vi "Arm Controller.vi"(8 "error in":errorcluster) -> ()   [LabVIEW 2018]
doc: "This VI executes continuously carrying out the current operation and responding to updates or new operations. It will often contain the timing or control code that is difficult to place directly in TeleOp. This VI generally opens all sensors and motors and isolates the rest of the robot code from knowing how the operations are carried out."
uses:
  <vilib>/Rock Robotics/WPI/Framework/Completion Status.ctl
  Arm Setpoints.ctl
  Arm Operations.ctl
  <vilib>/Rock Robotics/WPI/ThirdParty/Phoenix-LabVIEW/Motor Controller/Controls/CTRE_Phoenix_MotorControl_FeedbackDevice.ctl
  <vilib>/Rock Robotics/WPI/ThirdParty/Phoenix-LabVIEW/Motor Controller/Controls/CTRE_Phoenix_MotorControl_LimitSwitchSource_Local.ctl
  <vilib>/Rock Robotics/WPI/ThirdParty/Phoenix-LabVIEW/Motor Controller/Controls/CTRE_Phoenix_MotorControl_LimitSwitchNormal.ctl
  <vilib>/Rock Robotics/WPI/ThirdParty/Phoenix-LabVIEW/Motor Controller/Controls/CTRE_Phoenix_MotorControl_StatusFrameEnhanced.ctl
  <vilib>/Rock Robotics/WPI/ThirdParty/Phoenix-LabVIEW/Motor Controller/Controls/CTRE_Phoenix_MotorControl_VelocityMeasurementPeriod.ctl
  <vilib>/Rock Robotics/WPI/ThirdParty/Phoenix-LabVIEW/Motor Controller/Controls/CTRE_Phoenix_MotorControl_ControlMode.ctl
  <extravilib>/ChannelInstances/Lossy Stream-c(i32,i32,i32,i32)/Write With Abort.vi
  <extravilib>/ChannelInstances/Lossy Stream-c(i32,i32,i32,i32)/Read With Abort.vi
  <extravilib>/ChannelInstances/Lossy Stream-c(i32,i32,i32,i32)/Endpoint.vi
  <extravilib>/ChannelInstances/Lossy Stream-c(i32,i32,i32,i32)/EndpointRead.vi
  <extravilib>/ChannelInstances/Lossy Stream-c(i32,i32,i32,i32)/Instantiate.vi
  <extravilib>/ChannelInstances/Lossy Stream-c(i32,i32,i32,i32)/)Channel.vi
  <resource>/ChannelSupport/_ChannelSupport/WaitIfNeeded.vi
  <vilib>/Rock Robotics/WPI/ThirdParty/Phoenix-LabVIEW/Motor Controller/Get/CTRE_Phoenix_MotorController_GetSelectedSensorData.vi
  <extravilib>/ChannelInstances/Lossy Stream-c(i32,i32,i32,i32).lvlib
  <vilib>/Rock Robotics/Network Tables/NT Write Boolean.vi
panel:
  in  "F":dbl=11.9
  in  "D":dbl
  in  "I":dbl
  in  "P":dbl=8.0
  in  "Acceleration":i32=120
  in  "Cruise Velocity":i32=40
  in  "Gravity Compensator":dbl=0.038 format="%#_13g"
  in  "Interactive Values":T1
  out "Current\nCmd":string
  in  "Buttons":cluster{"Execute Cmd":bool, "Abort Cmd":bool}
  out "Command Timing":cluster{"Start Time (ms)":u32, "Iterations":i32}
  out "Status":T3
  # "Tip: It may be helpful to observe inputs and sensor values.\nYou may also want to display tuning or debugging controls."
  # "Interactive Command: You may fill in the settings for a command\nand schedule it with the Execute button. You can observe and abort\nany command while fine tuning the code for the controller."
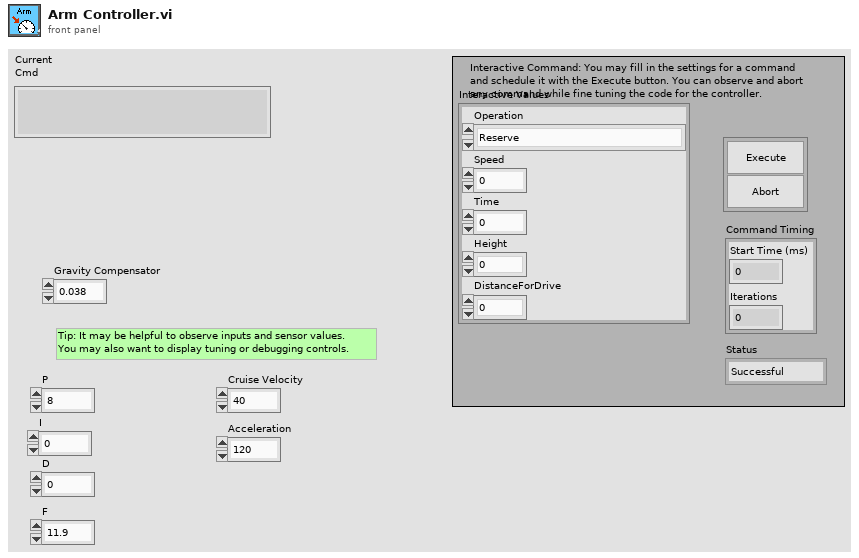
[diagram p1: front panel]
types:
  T1 = typedef "Arm Setpoints.ctl" = cluster{"Operation":T2, "Speed":dbl, "Time":dbl, "Height":dbl, "DistanceForDrive":dbl}
  T2 = typedef "Arm Operations.ctl" = enum16{"Reserve", "Read Current", "Immediate", "RaiseForTime", "GoToHeight", "StayAtHeight", "RaiseAfterTime", "RaiseAfterDriveAtDistance"}
  T3 = typedef "Completion Status.ctl" = enum16{"Successful", "Aborted", "Incomplete"}
  T4 = typedef "CTRE_Phoenix_MotorControl_VelocityMeasurementPeriod.ctl" = u16
  T5 = typedef "CTRE_Phoenix_MotorControl_StatusFrameEnhanced.ctl" = u16
  T6 = typedef "CTRE_Phoenix_MotorControl_LimitSwitchNormal.ctl" = enum16{"Normally Open", "Normally Closed", "Disabled"}
  T7 = typedef "CTRE_Phoenix_MotorControl_LimitSwitchSource_Local.ctl" = enum16{"Feedback Connector", "Remote Talon SRX", "Remote CANifier", "Deactivated"}
  T8 = typedef "CTRE_Phoenix_MotorControl_FeedbackDevice.ctl" = i8
  T9 = typedef "WPI_MotorControlDeviceRef.ctl" = cluster{"DeviceStatus":errorcluster, "Type":T10, "PWM":cluster{"PWM Channel":T11, "DeadBand":T12}, "CAN":cluster{"Device Number":u8, "SetOutput VI Ref":variant, "GetOutput VI Ref":variant, "Enable VI Ref":variant, "Disable VI Ref":variant, "Data":variant}, "Invert":bool, "DIO PWM":cluster{"PWM \"Enable\" Channel":T11, "DIOChannel":T13, "PWM Rate":dbl}}
  T10 = typedef "WPI_MotorControlType.ctl" = enum16{"PWM", "CAN", "DIO PWM"}
  T11 = typedef "FPGA_DIOPWMChannel.ctl" = enum8{"PWM 0", "PWM 1", "PWM 2", "PWM 3", "PWM 4", "PWM 5", "PWM 6", "PWM 7", "PWM 8", "PWM 9", "PWM MXP 0", "PWM MXP 1", "PWM MXP 2", "PWM MXP 3", "PWM MXP 4", "PWM MXP 5", "PWM MXP 6", "PWM MXP 7", "PWM MXP 8", "PWM MXP 9", "Invalid"}
  T12 = typedef "WPI_PWMDeadband.ctl" = cluster{"Name":string, "maxPositivePwm":i32, "minPositivePwm":i32, "centerPwm":i32, "maxNegativePwm":i32, "minNegativePwm":i32, "angularRange":u16}
  T13 = typedef "FPGA_DIOChannel.ctl" = enum8{"DIO 0", "DIO 1", "DIO 2", "DIO 3", "DIO 4", "DIO 5", "DIO 6", "DIO 7", "DIO 8", "DIO 9", "DIO MXP 0", "DIO MXP 1", "DIO MXP 2", "DIO MXP 3", "DIO MXP 4", "DIO MXP 5", "DIO MXP 6", "DIO MXP 7", "DIO MXP 8", "DIO MXP 9", "DIO MXP 10", "DIO MXP 11", "DIO MXP 12", "DIO MXP 13", "DIO MXP 14", "DIO MXP 15", "SPI Port CS1", "SPI Port CS2", "SPI Port CS3", "SPI Port MISO", "SPI Port MOSI", "Invalid"}
  T14 = typedef "Command Status Info.ctl" = cluster{"Name":string, "Status":T3, "notifier out":T15}
  T15 = typedef "Completion Notifier.ctl" = refnum<notifier>
  T16 = cluster{"Current Command":T1, "Command Timing":cluster{"Start Time (ms)":u32, "Iterations":i32}, "Command Arguments":cluster{"Command Info":T14, "Description":string, "Default Command":T1, "queue out":refnum<queue>, "Subsystem Name":string}}
  T17 = cluster{"Position":i32, "Velocity":i32, "Target Position":i32, "Target Velocity":i32}
  T18 = typedef "Lossy Stream-c(i32,i32,i32,i32).lvlib/)Channel.ctl" = refnum<queue>
  T19 = enum16{"DemandType_Neutral", "DemandType_AuxPID", "DemandType_ArbitraryFeedForward"}
  T20 = cluster{"Operation":T2, "Height":dbl, "DistanceForDrive":dbl, "Time":dbl}
  T21 = typedef "CTRE_Phoenix_MotorControl_ControlMode.ctl" = u16
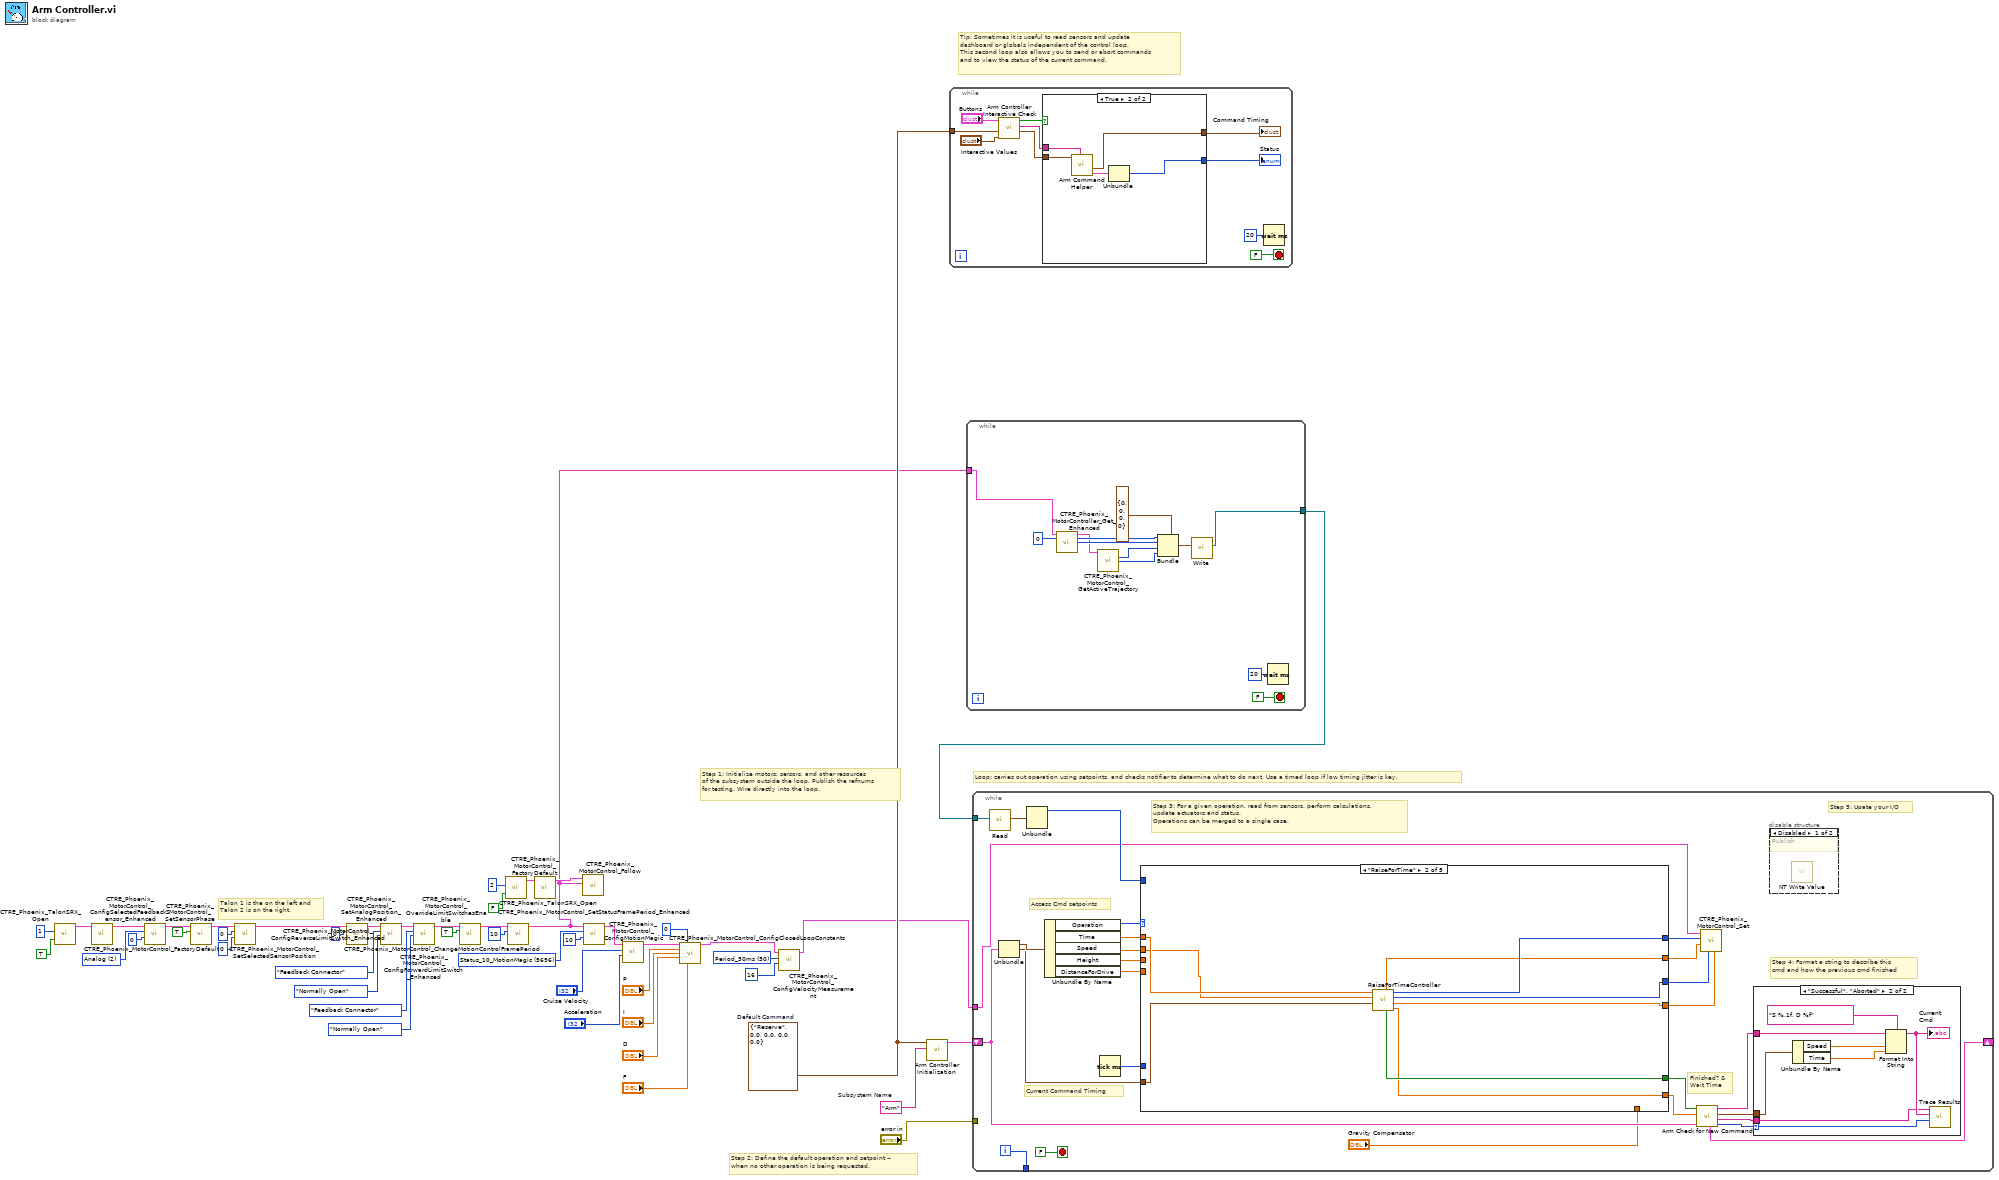
[diagram p0: block diagram]
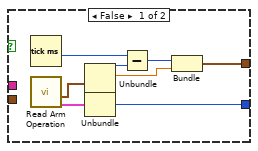
[diagram p2: hidden frame]
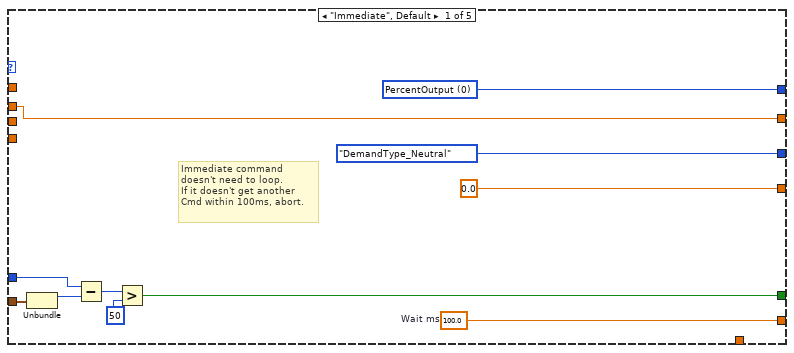
[diagram p5: hidden frame]
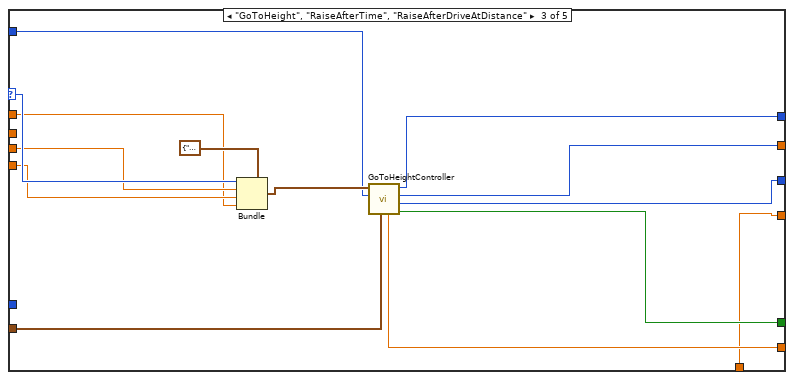
[diagram p6: hidden frame]
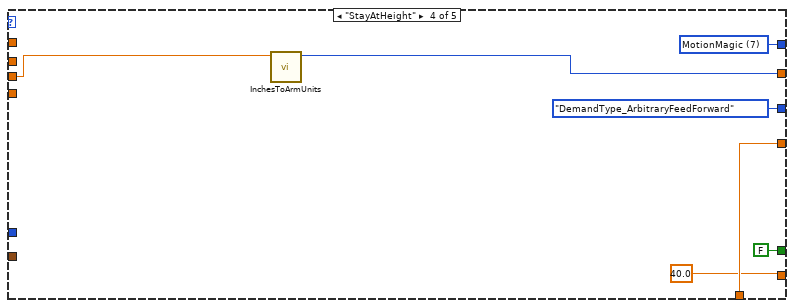
[diagram p7: hidden frame]
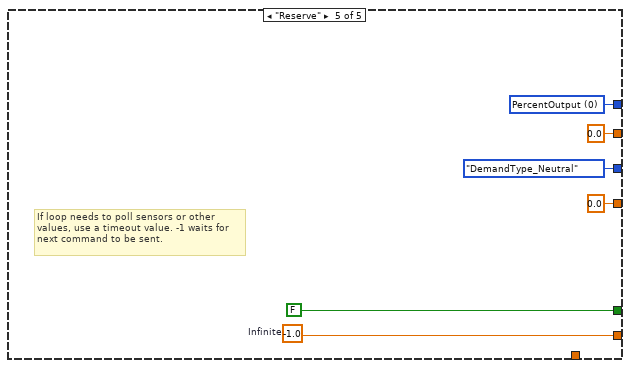
[diagram p8: hidden frame]
diagram:
  w13 = T4 50 items=["Period_1ms"=1, "Period_2ms"=2, "Period_5ms"=5, "Period_10ms"=10, "Period_20ms"=20, "Period_25ms"=25, "Period_50ms"=50, "Period_100ms"=100] ("Velocity Measurement Period")
  w21 = T5 5696 items=["Status_1_General"=5120, "Status_2_Feedback0"=5184, "Status_3_Quadrature"=5248, "Status_4_AinTempVbat"=5312, "Status_6_Misc"=5440, "Status_7_CommStatus"=5504, "Status_8_PulseWidth"=5568, "Status_9_MotProfBuffer"=5632, "Status_10_MotionMagic"=5696, "Status_11_UartGadgeteer"=5760, "Status_12_Feedback1"=5824, "Status_13_Base_PIDF0"=5888, "Status_14_Turn_PIDF1"=5952, "Status_15_FirmwareApiStatus"=6016] ("Status Frame")
  w38 = T8 2 items=["QuadEncoder"=0, "Analog"=2, "Tachometer"=4, "Pulse Width Encoded Position"=8, "Sensor Sum (S0 + S1)"=9, "Sensor Difference (D0 - D1)"=10, "Remote Source 0"=11, "Remote Source 1"=12, "Software Emulated"=15] ("Feedback Device")
  w45 = T1 {"Operation"=enum."Reserve", "Speed"=0.0, "Time"=0.0, "Height"=0.0, "DistanceForDrive"=0.0}  # Default Command
  w46 = "Arm"  # Subsystem Name
  # "Talon 1 is the on the left and\nTalon 2 is on the right."
  # "Tip: Sometimes it is useful to read sensors and update\ndashboard or globals independent of the control loop.\nThis second loop also allows you to send or abort commands\nand to view the status of the current command."
  # "Step 2: Define the default operation and setpoint --\nwhen no other operation is being requested."
  # "Step 1: Initialize motors, sersors, and other resources\nof the subsystem outside the loop. Publish the refnums\nfor testing. Wire directly into the loop."
  # "Loop: carries out operation using setpoints, and checks notifier to determine what to do next. Use a timed loop if low timing jitter is key."
  n1 = call <vilib>:"CTRE_Phoenix_TalonSRX_Open.vi"("Invert"=TRUE, "Device Number"=u8 1) -> ("CAN Talon SRX Ref"=w42:T9)  [unwired: 8 in, 1 out]
  n2 = call <vilib>:"CTRE_Phoenix_MotorControl_FactoryDefault.vi"("PhoenixMotorControlDevRef"=w42) -> ("PhoenixMotorControlDevRef"=w39:T9)  [unwired: 9 in, 1 out]
  n3 = call <vilib>:"CTRE_Phoenix_MotorControl_ConfigSelectedFeedbackSensor_Enhanced.vi"("pidLoopIdx"=0, "Feedback Device"=w38, "PhoenixMotorControlDevRef"=w39) -> ("PhoenixMotorControlDevRef"=w26:T9)  [unwired: 7 in, 1 out]
  n4 = call <vilib>:"CTRE_Phoenix_MotorControl_SetSensorPhase.vi"("PhaseSensor"=TRUE, "PhoenixMotorControlDevRef"=w26) -> ("PhoenixMotorControlDevRef"=w24:T9)  [unwired: 8 in, 1 out]
  n5 = call <vilib>:"CTRE_Phoenix_MotorControl_SetSelectedSensorPosition.vi"("pidLoopIdx"=u32 0, "New Sensor Position"=0, "PhoenixMotorControlDevRef"=w24) -> ("PhoenixMotorControlDevRef"=w17:T9)  [unwired: 7 in, 1 out]
  n6 = call <vilib>:"CTRE_Phoenix_MotorControl_SetAnalogPosition_Enhanced.vi"("New Position"=0, "PhoenixMotorControlDevRef"=w17) -> ("PhoenixMotorControlDevRef"=w16:T9)  [unwired: 8 in, 1 out]
  n7 = call <vilib>:"CTRE_Phoenix_MotorControl_ConfigReverseLimitSwitch_Enhanced.vi"("PhoenixMotorControlDevRef"=w16, "Limit Switch Source"=CTRE_Phoenix_MotorControl_LimitSwitchSource_Local."Feedback Connector", "NormallyOpenOrClosed"=CTRE_Phoenix_MotorControl_LimitSwitchNormal."Normally Open") -> ("PhoenixMotorControlDevRef"=w34:T9)  [unwired: 11 in, 1 out]
  n8 = call <vilib>:"CTRE_Phoenix_MotorControl_ConfigForwardLimitSwitch_Enhanced.vi"("PhoenixMotorControlDevRef"=w34, "Limit Switch Source"=CTRE_Phoenix_MotorControl_LimitSwitchSource_Local."Feedback Connector", "NormallyOpenOrClosed"=CTRE_Phoenix_MotorControl_LimitSwitchNormal."Normally Open") -> ("PhoenixMotorControlDevRef"=w29:T9)  [unwired: 11 in, 1 out]
  n9 = call <vilib>:"CTRE_Phoenix_MotorControl_OverrideLimitSwitchesEnable.vi"("PhoenixMotorControlDevRef"=w29, "Override Limit Switch Enable?"=TRUE) -> ("PhoenixMotorControlDevRef"=w19:T9)  [unwired: 12 in, 1 out]
  n10 = call <vilib>:"CTRE_Phoenix_TalonSRX_Open.vi"("Invert"=FALSE, "Device Number"=u8 2) -> ("CAN Talon SRX Ref"=w40:T9)  [unwired: 8 in, 1 out]
  n11 = call <vilib>:"CTRE_Phoenix_MotorControl_ChangeMotionControlFramePeriod.vi"("periodMs"=10, "PhoenixMotorControlDevRef"=w19) -> ("PhoenixMotorControlDevRef"=w2:T9)  [unwired: 8 in, 1 out]
  n12 = call <vilib>:"CTRE_Phoenix_MotorControl_FactoryDefault.vi"("PhoenixMotorControlDevRef"=w40) -> ("PhoenixMotorControlDevRef"=w27:T9)  [unwired: 9 in, 1 out]
  n13 = call <vilib>:"CTRE_Phoenix_MotorControl_Follow.vi"("Master Controller to Follow"=w2, "PhoenixMotorControlDevRef"=w27) -> ()  [unwired: 8 in, 2 out]
  n14 = call <vilib>:"CTRE_Phoenix_MotorControl_SetStatusFramePeriod_Enhanced.vi"("periodMs"=10, "Status Frame"=w21, "PhoenixMotorControlDevRef"=w2) -> ("PhoenixMotorControlDevRef"=w4:T9)  [unwired: 7 in, 1 out]
  n15 = call <vilib>:"CTRE_Phoenix_MotorControl_ConfigMotionMagic.vi"("Acceleration"="Acceleration", "Cruise Velocity"="Cruise Velocity", "PhoenixMotorControlDevRef"=w4) -> ("PhoenixMotorControlDevRef"=w7:T9)  [unwired: 7 in, 1 out]
  n16 = call <vilib>:"CTRE_Phoenix_MotorControl_ConfigClosedLoopConstants.vi"("PhoenixMotorControlDevRef"=w7, "slotIdx"=0, "P"="P", "I"="I", "D"="D", "F"="F") -> ("PhoenixMotorControlDevRef"=w3:T9)  [unwired: 8 in, 1 out]
  n17 = call <vilib>:"CTRE_Phoenix_MotorControl_ConfigVelocityMeasurement.vi"("Window Size"=16, "Velocity Measurement Period"=w13, "PhoenixMotorControlDevRef"=w3) -> ("PhoenixMotorControlDevRef"=w12:T9)  [unwired: 7 in, 1 out]
  n18 = call "Arm Controller Initialization.vi"("Subsystem Name"=w46, "Default Command"=w45) -> ("Current Command"=w47:T16)  [unwired: 9 in]
  n19 = while {
    tunnel: w45 -> [w55]
    stop <- FALSE stop-if-true
    n20 = call "Arm Controller Interactive Check.vi"("Interactive Command in"="Interactive Values", "Default Command"=w55, "Buttons"="Buttons") -> ("Interactive Command out"=w52:T1, "Trace String"=w53:string, "Schedule"=w54:bool)  [unwired: 6 in]
    n21 = case shown="True" w54 {
      tunnel: [w66 w71] -> w51
      tunnel: w52 -> [_ w69]
      tunnel: [w62 w67] -> w50
      tunnel: w53 -> [_ w70]
      frame False {
        n22 = Tick Count (ms)() -> (millisecond timer value=w61:u32)
        n23 = call "Read Arm Operation.vi"() -> ("Command Info"=w59:T14, "SubSystem Data"=w60:T1)  [unwired: 9 in, 1 out]
        n24 = Unbundle(w60) -> ("Operation"=w65:T2, "Speed"=w63:dbl)  [unwired: 3 out]
        n25 = Unbundle(w59) -> ("Status"=w66:T3)  [unwired: 2 out]
        n26 = Subtract(x=w61, y=w65) -> (x-y=w64:u32)
        n27 = Bundle(w64, "Speed"=w63) -> (w62:cluster{u32, "Speed":dbl})  [unwired: 1 in]
      }
      frame True {
        n28 = call "Arm Command Helper.vi"("Description"=w70, "SubSystem Data"=w69) -> ("Command Info Out"=w68:T14, "Command Timing"=w67:cluster{"Start Time (ms)":u32, "Iterations":i32})  [unwired: 7 in, 1 out]
        n29 = Unbundle(w68) -> ("Status"=w71:T3)  [unwired: 2 out]
      }
    }
    "Status" <- w51
    "Command Timing" <- w50
    n30 = Wait (ms)(milliseconds to wait=u32 20) -> ()  [unwired: 1 out]
  }
  n31 = while {
    tunnel: w2 -> [w73]
    tunnel: [w72] -> w44
    stop <- FALSE stop-if-true
    n32 = call-poly <vilib>:"CTRE_Phoenix_MotorController_Get_Enhanced.vi"("PhoenixMotorControlDevRef"=w73, "pidLoopIdx"=u32 0) -> ("PhoenixMotorControlDevRef"=w75:T9, "Position (Raw Sensor Units)"=w80:i32, "Velocity (Raw Sensor Units per 100 ms)"=w79:i32)  [unwired: 10 in, 1 out]
    n33 = call <vilib>:"CTRE_Phoenix_MotorControl_GetActiveTrajectory.vi"("PhoenixMotorControlDevRef"=w75) -> ("Position (Sensor Units)"=w77:i32, "Velocity (Sensor Units per 100 ms)"=w74:i32)  [unwired: 10 in, 3 out]
    n34 = Bundle(cluster=T17 {"Position"=0, "Velocity"=0, "Target Position"=0, "Target Velocity"=0} ("Sensor Data"), "Position"=w80, "Velocity"=w79, "Target Position"=w77, "Target Velocity"=w74) -> (w76:T17)
    n35 = call <extravilib>:"Write.vi"("element"=w76) -> ("channel"=w72:T18)  [unwired: 8 in, 2 out]
    n36 = Wait (ms)(milliseconds to wait=u32 20) -> ()  [unwired: 1 out]
  }
  n37 = while {
    shift-right: [w102] -> _
    shift-left: w47 -> [w97]
    tunnel: [w109] -> _
    tunnel: "error in" -> [_]
    tunnel: w12 -> [w86]
    tunnel: w44 -> [w85]
    i -> [w109]
    stop <- FALSE stop-if-true
    # "Step 5: Upate your I/O"
    # "Step 4: Format a string to describe this\ncmd and how the previous cmd finished"
    # "Current Command Timing"
    # "Access Cmd setpoints"
    # "Finished? &\nWait Time"
    # "Step 3: For a given operation, read from sensors, perform calculations,\nupdate actuators and status.\nOperations can be merged to a single case."
    n38 = call <extravilib>:"Read.vi"("channel"=w85) -> ("element"=w84:T17)  [unwired: 5 in, 5 out]
    n39 = Unbundle(w97) -> ("Current Command"=w108:T1, "Command Timing"=w104:cluster{"Start Time (ms)":u32, "Iterations":i32})  [unwired: 1 out]
    n40 = Unbundle(w84) -> ("Position"=w89:i32)  [unwired: 3 out]
    n41 = Unbundle By Name(w108) -> ("Operation"=w107:T2, "Time"=w106:dbl, "Speed"=w103:dbl, "Height"=w93:dbl, "DistanceForDrive"=w92:dbl)
    n42 = Tick Count (ms)() -> (millisecond timer value=w105:u32)
    n43 = case shown="\"RaiseForTime\"" w107 {
      selector: w107 -> [_ _ w145 _ _]
      tunnel: [w129 w131 w152 40.0 w165] -> w91
      tunnel: [w123 w136 w151 FALSE ("ignore previous (F)") FALSE ("ignore previous (F)")] -> w90
      tunnel: w104 -> [w125 w138 w147 _ _]
      tunnel: w106 -> [_ w137 w140 _ _]
      tunnel: w105 -> [w124 _ _ _ _]
      tunnel: w103 -> [w122 w132 _ _ _]
      tunnel: [w121 w135 w148 w157 w160] -> w96
      tunnel: [w122 w130 w149 w155 0.0 ("Speed")] -> w95
      tunnel: [T19."DemandType_Neutral" ("DemandType") w134 w150 T19."DemandType_ArbitraryFeedForward" ("DemandType") T19."DemandType_Neutral" ("DemandType")] -> w94
      tunnel: [0.0 ("Demand1") w133 w146 w159 0.0 ("Gravity Compensator")] -> w87
      tunnel: w93 -> [_ _ w142 w156 _]
      tunnel: w92 -> [_ _ w141 _ _]
      tunnel: w89 -> [_ _ w139 _ _]
      tunnel: "Gravity Compensator" -> [_ _ w146 w159 _]
      frame "Immediate", Default {
        w121 = T21 0 items=["PercentOutput"=0, "Position"=1, "Velocity"=2, "Current"=3, "Follower"=5, "MotionProfile"=6, "MotionMagic"=7, "MotionProfileArc"=10, "Disabled"=15] ("Control Mode")
        w129 = 100.0  # Wait ms
        # "Immediate command\ndoesn't need to loop.\nIf it doesn't get another\nCmd within 100ms, abort."
        n44 = Unbundle(w125) -> ("Start Time (ms)"=w128:u32)  [unwired: 1 out]
        n45 = Subtract(x=w124, y=w128) -> (x-y=w127:u32)
        n46 = Greater?(x=w127, y=u8 50 ("Left Motor")) -> (0:w123:bool)
      }
      frame "RaiseForTime" {
        n47 = call "RaiseForTimeController.vi"("Command Timing"=w138, "Speed"=w132, "Time"=w137) -> ("Delay"=w131:dbl, "Demand1"=w133:dbl, "DemandType"=w134:T19, "Control Mode"=w135:T21, "Done"=w136:bool, "SpeedOut"=w130:dbl)  [unwired: 3 in]
      }
      frame "GoToHeight", "RaiseAfterTime", "RaiseAfterDriveAtDistance" {
        n48 = Bundle(cluster=T20 {"Operation"=enum."Reserve", "Height"=0.0, "DistanceForDrive"=0.0, "Time"=0.0} ("Setpoints"), "Operation"=w145, "Height"=w142, "DistanceForDrive"=w141, "Time"=w140) -> (w143:T20)
        n49 = call "GoToHeightController.vi"("Command Timing"=w147, "Position"=w139, "Setpoints"=w143) -> ("Done"=w151:bool, "DemandType"=w150:T19, "Output"=w149:i32, "Control Mode"=w148:T21, "Delay"=w152:dbl)  [unwired: 4 in]
      }
      frame "StayAtHeight" {
        w157 = T21 7 items=["PercentOutput"=0, "Position"=1, "Velocity"=2, "Current"=3, "Follower"=5, "MotionProfile"=6, "MotionMagic"=7, "MotionProfileArc"=10, "Disabled"=15] ("Control Mode")
        n50 = call "InchesToArmUnits.vi"("Inches"=w156) -> ("Sensor Units"=w155:i32)  [unwired: 10 in]
      }
      frame "Reserve" {
        w160 = T21 0 items=["PercentOutput"=0, "Position"=1, "Velocity"=2, "Current"=3, "Follower"=5, "MotionProfile"=6, "MotionMagic"=7, "MotionProfileArc"=10, "Disabled"=15] ("Control Mode")
        w165 = -1.0  # Infinite
        # "If loop needs to poll sensors or other\nvalues, use a timeout value. -1 waits for\nnext command to be sent."
      }
    }
    n51 = call "Arm Check for New Command.vi"("Current Command"=w97, "Wait time (ms)"=w91, "Finished?"=w90) -> ("Completion"=w98:T3, "Subsystem Name"=w99:string, "Current Command"=w100:T1, "Initial Trace String"=w101:string, "NextCommand"=w102:T16)  [unwired: 4 in]
    n52 = call <vilib>:"CTRE_Phoenix_MotorControl_Set.vi"("Demand1"=w87, "DemandType"=w94, "Output"=w95, "Control Mode"=w96, "PhoenixMotorControlDevRef"=w86) -> ()  [unwired: 5 in, 2 out]
    n53 = case shown="\"Successful\", \"Aborted\"" w98 {
      selector: w98 -> [_ w118]
      tunnel: w101 -> [_ w114]
      tunnel: w100 -> [_ w115]
      tunnel: w99 -> [_ w111]
      frame "Incomplete", Default {
        # "Continuing current command"
      }
      frame "Successful", "Aborted" {
        # "Report and setup for next command"
        n54 = Unbundle By Name(w115) -> ("Speed"=w117:dbl, "Time"=w112:dbl)
        n55 = Format Into String(format string="S %.1f, D %f", initial string=w114, w117, w112) -> (resulting string=w113:string)  [unwired: 1 in, 1 out]
        "Current\nCmd" <- w113
        n56 = call <vilib>:"Trace Results.vi"("Status of previous command"=w118, "Description"=w113, "Subsystem"=w111) -> ()  [unwired: 9 in]
      }
    }
    n57 = disable-structure shown="Disabled" {
      frame Disabled {
        # "Publish"
        n58 = call-poly <vilib>:"NT Write Value.vi"() -> ()  [unwired: 11 in, 1 out]
      }
      frame Enabled {
      }
    }
  }
